vi "rotate PID.vi"(5 "output range":cluster{"output high":dbl, "output low":dbl}={"output high"=100.0, "output low"=-100.0} {"output low" format="%.2f"; "output high" format="%.2f"}, 6 "s":bool, 7 "PID":cluster{"Kp":dbl, "Ki":dbl, "Kd":dbl}, 8 "dt (s)":dbl=-1.0 format="%.3f", 9 "Processer":dbl, 10 "setpoint":dbl) -> (0 "e(t)":dbl, 1 "out":dbl)   [LabVIEW 2019]
uses:
  <vilib>/addons/control/pid/pid.llb/PID (DBL).vi
  <vilib>/addons/control/pid/NI_PID_pid.lvlib
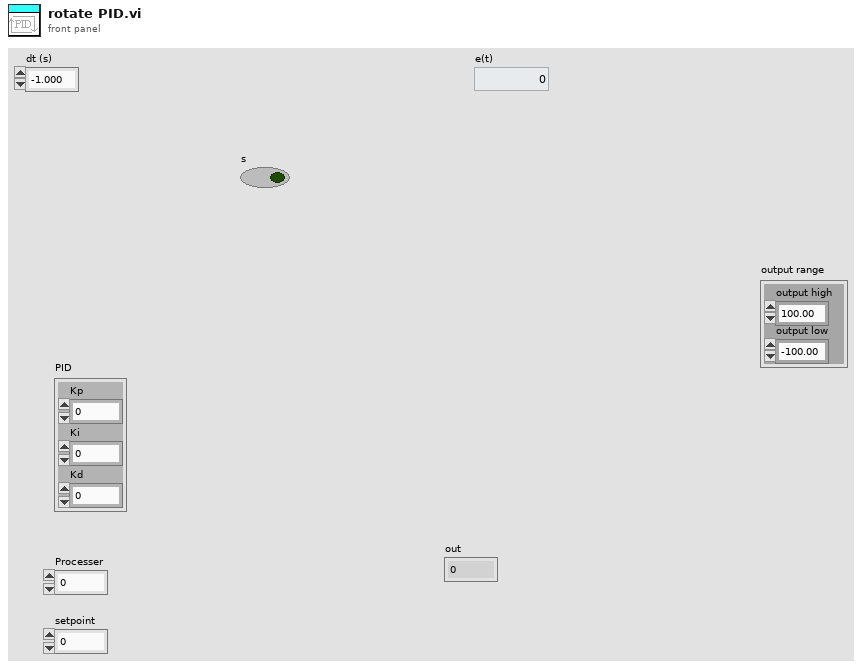
[diagram p1: front panel]
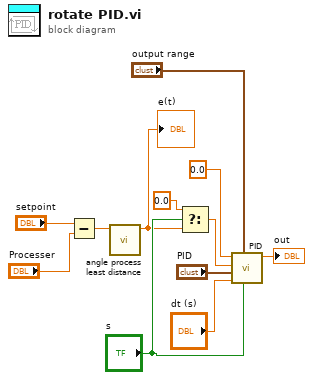
[diagram p0: block diagram]
diagram:
  n1 = Subtract(x="setpoint", y="Processer") -> (x-y=w9:dbl)
  n2 = call "angle process least distance.vi"("Numeric in"=w9) -> ("Numeric out"=w1:dbl)  [unwired: 10 in]
  "e(t)" <- w1
  n3 = Select(t=0.0, s="s", f=w1) -> (s? t:f=w3:dbl)
  n4 = call-poly <vilib>:"PID.vi"("reinitialize? (F)"="s", "output range"="output range", "dt (s)"="dt (s)", "PID gains"="PID", "process variable"=w3, "setpoint"=0.0) -> ("output"=→"out":dbl)  [unwired: 4 in, 1 out]
